vi "Read raDecParameters.vi"(8 "error in (no error)":errorcluster, 11 "RADecTarget in":refnum<class "RADecTarget.lvclass">) -> (0 "error out":errorcluster, 2 "RADecParameters.lvclass":refnum<class "RADecParameters.lvclass">, 3 "RADecTarget out":refnum<class "RADecTarget.lvclass">)   [LabVIEW 2022 SP3, in "TCSDataDefinitions.lvlib" / "TCSCommand.lvlib" / "TargetConfiguration.lvlib" / "Target.lvlib" / "FixedTarget.lvlib" / "RADecTarget.lvclass"]
uses:
  RADecTarget.lvclass
  RADecParameters/RADecParameters.lvclass
  RADecTarget.lvclass/RADecTarget.ctl
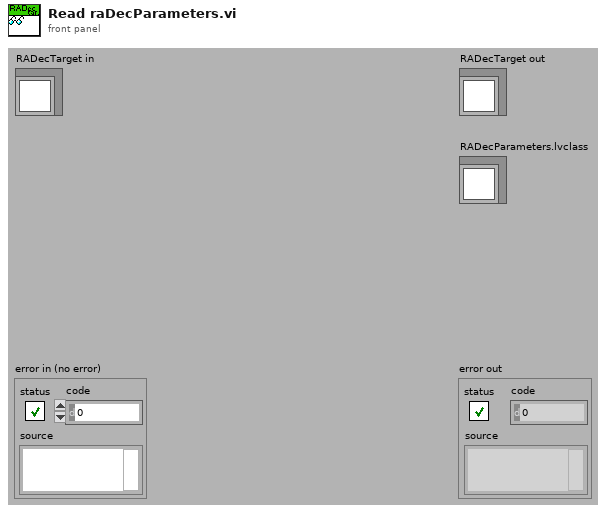
[diagram p1: front panel]
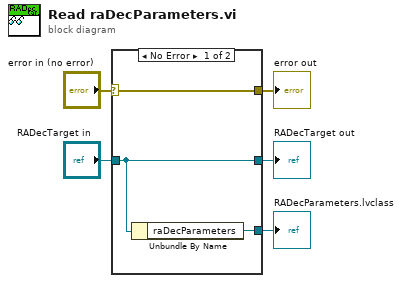
[diagram p0: block diagram]
diagram:
  n1 = case shown="No Error" "error in (no error)" {
    selector: "error in (no error)" -> [w8 w9]
    tunnel: [w8 w9] -> w4
    tunnel: [w7 w10] -> w2
    tunnel: "RADecTarget in" -> [w7 w10]
    tunnel: [w6 _] -> w1
    frame No Error {
      n2 = Unbundle By Name(w7) -> ("raDecParameters"=w6:refnum<class "RADecParameters.lvclass">)
    }
    frame Error {
    }
  }
  "error out" <- w4
  "RADecTarget out" <- w2
  "RADecParameters.lvclass" <- w1
